vi "q2 two while loops parallel.vi"() -> ()   [LabVIEW 2025]
panel:
  in  "threshold":dbl
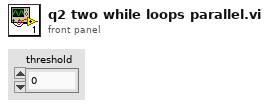
[diagram p1: front panel]
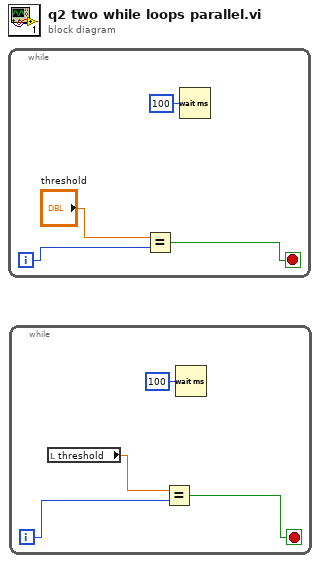
[diagram p0: block diagram]
diagram:
  n1 = while {
    i -> [w2]
    stop <- w1 stop-if-true
    n2 = Equal?(x="threshold", y=w2) -> (x = y?=w1:bool)
    n3 = Wait (ms)(milliseconds to wait=100) -> ()  [unwired: 1 out]
  }
  n4 = while {
    i -> [w5]
    stop <- w7 stop-if-true
    n5 = local read "threshold"() -> (w6:dbl)
    n6 = Equal?(x=w6, y=w5) -> (x = y?=w7:bool)
    n7 = Wait (ms)(milliseconds to wait=100) -> ()  [unwired: 1 out]
  }
